vi "Set Pixel (Grey).vi"(4 "Error":string, 5 "Value":u8, 6 "Y":i32, 7 "X":i32, 8 "Image":T1={"Image ID"=0, "Channel ID"=-1}) -> (0 "Error":string, 3 "Image":T1={"Image ID"=0, "Channel ID"=-1})   [LabVIEW 2011, in "labvvis.lvlib"]
doc: "Changes the value of the pixel in Image, at position (X, Y) to Value. This VI is applicable for both grey-scale images and single-channel images (like Red channel, Green channel and so on)."
uses:
  <userlib>/labvvis/labvvis.lvlib
  <userlib>/labvvis/VVIS Image.ctl
  labvvis.framework
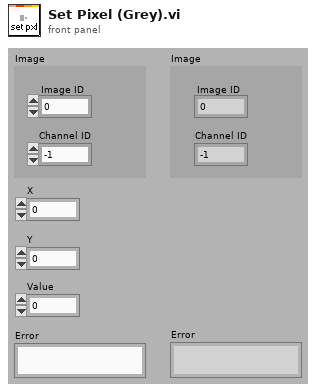
[diagram p1: front panel]
types:
  T1 = typedef "labvvis.lvlib/VVIS Image.ctl" = cluster{"Image ID":i16, "Channel ID":i16}
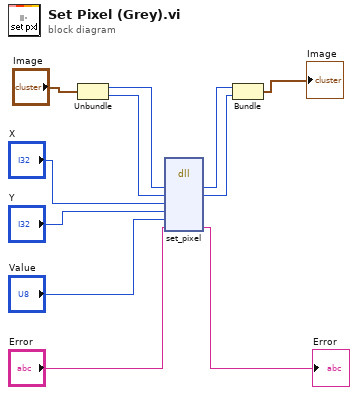
[diagram p0: block diagram]
diagram:
  n1 = Unbundle("Image") -> ("Image ID"=w9:i16, "Channel ID"=w8:i16)
  n2 = dll-call lib="labvvis.framework" fn="set_pixel"("out"=w9, "cid"=w8, "x"="X", "y"="Y", "value"="Value", "error"="Error") -> ("out"=w10:i16, "cid"=w2:i16, "error"=→"Error":string)  [unwired: 7 in, 2 out]
  n3 = Bundle("out"=w10, "cid"=w2) -> (→"Image":cluster{"out":i16, "cid":i16})  [unwired: 1 in]
